vi "Get all sensor data.vi"(6 "error in":errorcluster, 9 "Data Highway In":T1={"New Image"=refnum, "Session Out"="", "LIDAR VISA Name"="", "Phidget Device Out"=0, "Lidar Data"=[], "polar attributes"={"maximum"=0.0, "minimum"=0.0, "clip to min"=FALSE, "log?(F)"=FALSE, "grid color"=6710886, "plot color"=65280, "fmt and prec"={"format"=enum."Decimal", "precision"=0}, "visible section"=8}, "Debug Statement"="", "Servo Angles"={"Angle X"=0.0, "Angle Y"=0.0}} {"polar attributes"."minimum" format="%0.2f"; "polar attributes"."maximum" format="%0.2f"}) -> (0 "error out":errorcluster, 3 "Data Highway Out":T1={"New Image"=refnum, "Session Out"="", "LIDAR VISA Name"="", "Phidget Device Out"=0, "Lidar Data"=[], "polar attributes"={"maximum"=0.0, "minimum"=0.0, "clip to min"=FALSE, "log?(F)"=FALSE, "grid color"=6710886, "plot color"=65280, "fmt and prec"={"format"=enum."Decimal", "precision"=0}, "visible section"=8}, "Debug Statement"="", "Servo Angles"={"Angle X"=0.0, "Angle Y"=0.0}} {"polar attributes"."minimum" format="%0.2f"; "polar attributes"."maximum" format="%0.2f"})   [LabVIEW 2014]
uses:
  controls/Data.ctl
  <vilib>/vision/Image Controls.llb/IMAQ Image.ctl
  <vilib>/userdefined/High Color/IMAQdx.ctl
  Program Files (x86)/National Instruments/LabVIEW 2014/instr.lib/Hokuyo URG Series/Hokuyo URG Series.lvlib
  <vilib>/vision/driver/NI_Vision_Acquisition_Software.lvlib
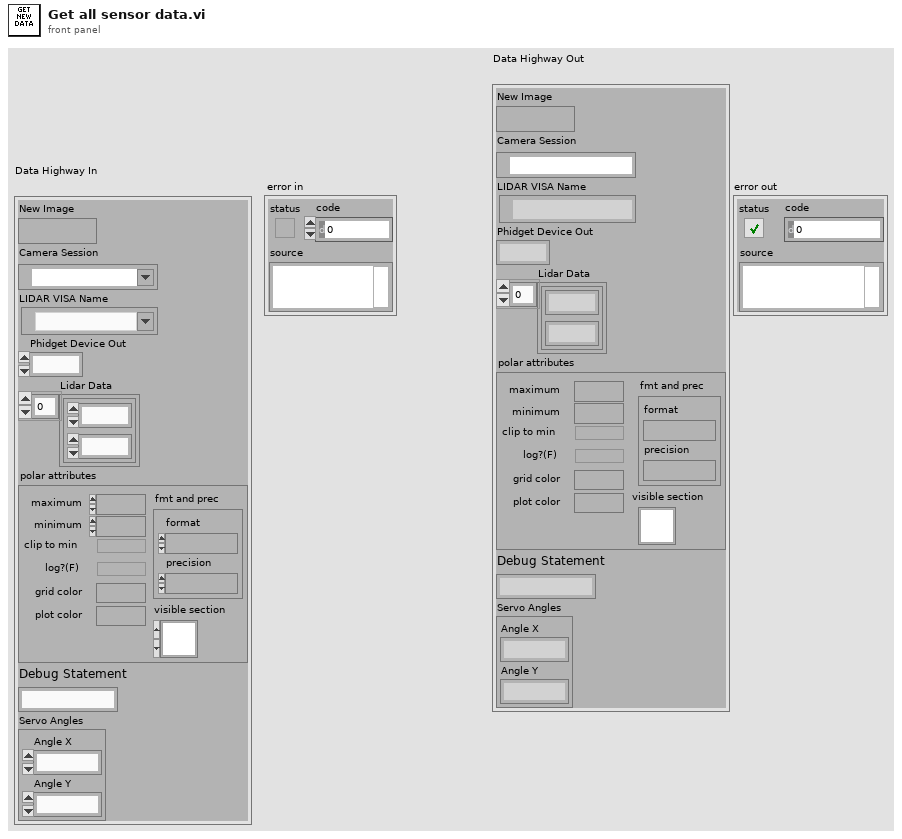
[diagram p1: front panel]
types:
  T1 = typedef "Data.ctl" = cluster{"New Image":T2, "Session Out":T3, "LIDAR VISA Name":refnum<visa-resource-name>, "Phidget Device Out":i32, "Lidar Data":cluster{dbl, dbl}[], "polar attributes":cluster{"maximum":dbl, "minimum":dbl, "clip to min":bool, "log?(F)":bool, "grid color":u32, "plot color":u32, "fmt and prec":cluster{"format":enum8{"Decimal", "Scientific", "Engineering", "Binary", "Octal", "Hex"}, "precision":u8}, "visible section":u16}, "Debug Statement":string, "Servo Angles":cluster{"Angle X":dbl, "Angle Y":dbl}}
  T2 = typedef "IMAQ Image.ctl" = refnum<image>
  T3 = typedef "IMAQdx.ctl" = refnum<k21>
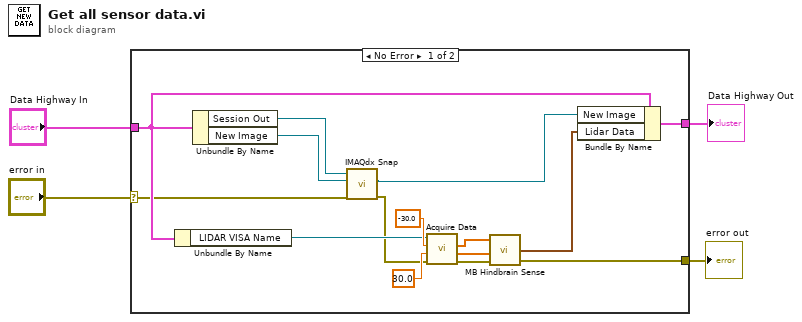
[diagram p0: block diagram]
diagram:
  n1 = case shown="No Error" "error in" {
    selector: "error in" -> [w6 w20]
    tunnel: [w13 w21] -> w4
    tunnel: "Data Highway In" -> [w12 w21]
    tunnel: [w10 w20] -> w2
    frame No Error {
      n2 = Unbundle By Name(w12) -> ("LIDAR VISA Name"=w14:refnum<visa-resource-name>)
      n3 = Unbundle By Name(w12) -> ("Session Out"=w9:T3, "New Image"=w8:T2)
      n4 = call <vilib>:"IMAQdx Snap.vi"("error in"=w6, "Image In"=w8, "Session In"=w9) -> ("error out"=w7:errorcluster, "Image Out"=w5:T2)  [unwired: 6 in, 1 out]
      n5 = call "Acquire Data.vi"("error in (no error)"=w7, "End Point (120°)"=30.0, "Start Point (-120°)"=-30.0, "VISA resource name"=w14) -> ("error out"=w11:errorcluster, "Direction"=w16:dbl[], "Magnitude"=w17:dbl[])  [unwired: 4 in, 1 out]
      n6 = call "MB Hindbrain Sense.vi"("error in"=w11, "Direction"=w16, "Magnitude"=w17) -> ("error out"=w10:errorcluster, "Lidar Data"=w15:cluster{dbl, dbl}[])  [unwired: 1 in]
      n7 = Bundle By Name(cluster=w12, "New Image"=w5, "Lidar Data"=w15) -> (w13:T1)
    }
    frame Error {
    }
  }
  "Data Highway Out" <- w4
  "error out" <- w2
